vi "Logging.vi"(6 "TDMS Refnum in":refnum<k34>, 8 "Signals to log":dbl[][](array[numeric]), 9 "Controller output":dbl, 10 "Log?":dbl, 11 "error in (no error)":errorcluster) -> (3 "error out":errorcluster, 4 "TDMS Refnum out":refnum<k34>)   [LabVIEW 2016]
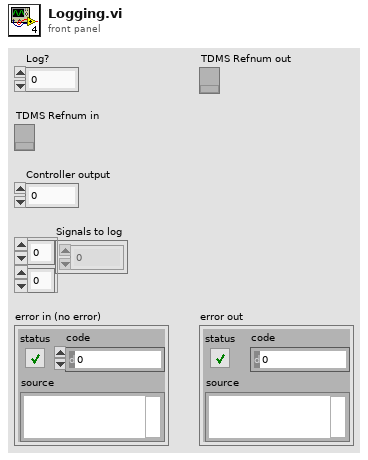
[diagram p1: front panel]
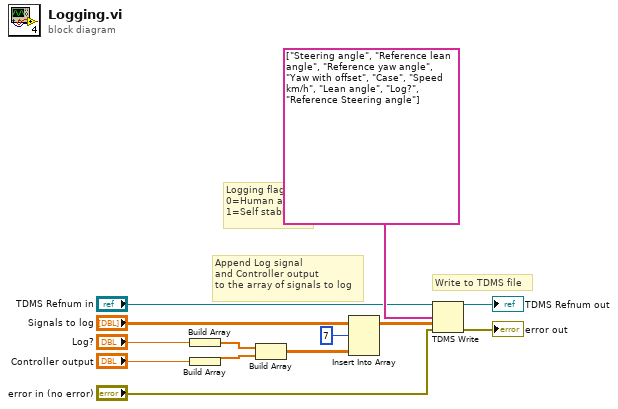
[diagram p0: block diagram]
diagram:
  # "Write to TDMS file"
  # "Append Log signal\nand Controller output\nto the array of signals to log"
  # "Logging flag\n0=Human aid\n1=Self stabilsing"
  n1 = Build Array("Log?") -> (w6:dbl[])
  n2 = Build Array("Controller output") -> (w7:dbl[])
  n3 = Build Array(w6, w7) -> (w9:dbl[][])
  n4 = Insert Into Array(array="Signals to log", index (row)=7, new element=w9) -> (w10:dbl[][])  [unwired: 1 in]
  n5 = TDMS Write(0:"TDMS Refnum in", 7:string[] ["Steering angle", "Reference lean angle", "Reference yaw angle", "Yaw with offset", "Case", "Speed km/h", "Lean angle", "Log?", "Reference Steering angle"] ("channel name(s) in (Untitled)"), 9:w10, 11:"error in (no error)") -> (4:→"TDMS Refnum out":refnum<k34>, 15:→"error out":errorcluster)  [unwired: 2 in, 2 out]
